vi "Get Scanner (basic).vi"(8 "error in (no error)":errorcluster, 11 "Pulse Generator in":refnum<class "Pulse Generator.lvclass">) -> (0 "error out":errorcluster, 2 "Pulse Gen Basic Scanner out":refnum<class "Scanner.lvclass">)   [LabVIEW 2009, in "Pulse Generator.lvclass"]
doc: "(Dynamic) Returns the default Scanner object that scans over this Scannable. (Note that a Scannable may have multiple Scanners associated with it.) A Scanner is an analogue to an Iterator class in other languages."
uses:
  Pulse Generator.lvclass
  Scanners/Scanner/Scanner.lvclass
  Scanners/Pulse Gen Basic Scan/Pulse Gen Basic Scan.lvclass
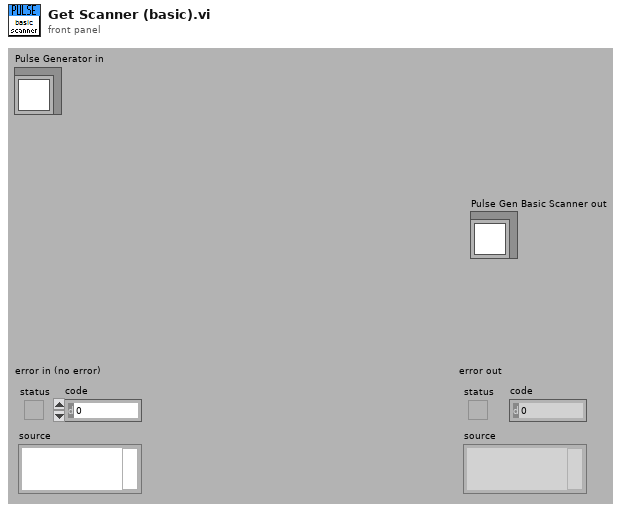
[diagram p1: front panel]
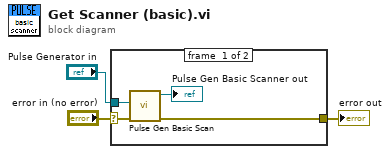
[diagram p0: block diagram]
diagram:
  n1 = case shown="No Error" "error in (no error)" {
    selector: "error in (no error)" -> [w5 w8]
    tunnel: [w6 w8] -> w2
    tunnel: "Pulse Generator in" -> [w4 _]
    frame #0 {
      n2 = call "Pulse Gen Basic Scan.vi"("error in (no error)"=w5, "Pulse Generator.lvclass"=w4) -> ("error out"=w6:errorcluster, "Pulse Gen Basic Scan out"=→"Pulse Gen Basic Scanner out":refnum<class "Pulse Gen Basic Scan.lvclass">)  [unwired: 8 in]
    }
    frame #1 {
    }
  }
  "error out" <- w2
